vi "FRCts20_Backend_Test_ClosedRequests.vi"(8 "error in (no error)":errorcluster, 11 "Event Name":string) -> (0 "error out":errorcluster, 1 "Time (ms)":u32, 2 "Status":string, 5 "Success":bool)   [LabVIEW 2014, in "FRCts20_Backend_TestCode.lvlib"]
uses:
  FRCts20_Backend_TestCode.lvlib
  FRCts20_Backend_API/FRCts20_Backend_API_ClosedRequests.ctl
  FRCts20_Backend_API/FRCts20_Backend_API_Command_ClosedRequests.ctl
  FRCts20_Backend_API/FRCts20_Backend_API_ClosedRequests.vi
  FRCts20_Backend_API/FRCts20_Backend_API.lvlib
panel:
  out "DataOut":T1
  # "368\n381"
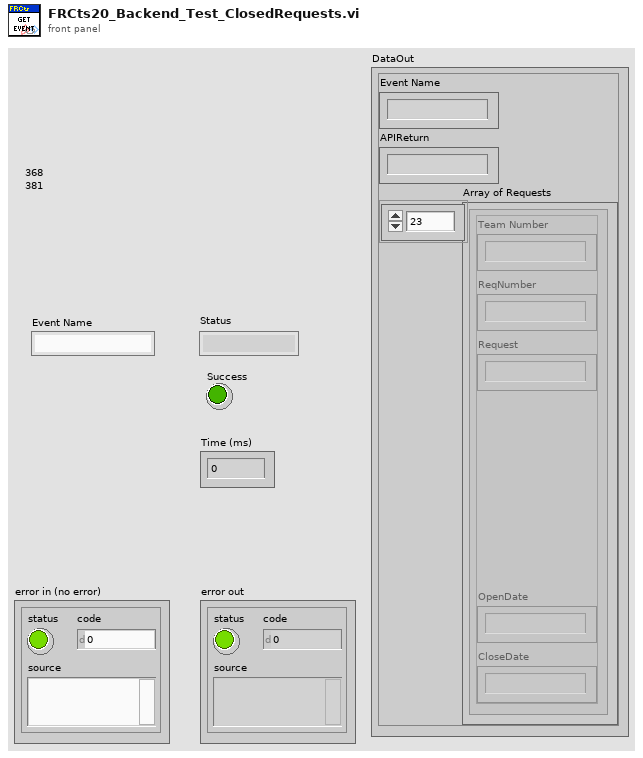
[diagram p1: front panel]
types:
  T1 = typedef "FRCts20_Backend_API.lvlib/FRCts20_Backend_API_ClosedRequests.ctl" = cluster{"Event Name":string, "APIReturn":string, "Array of Requests":cluster{"Team Number":string, "ReqNumber":string, "Request":string, "OpenDate":string, "CloseDate":string}[]}
  T2 = typedef "FRCts20_Backend_API.lvlib/FRCts20_Backend_API_Command_ClosedRequests.ctl" = string
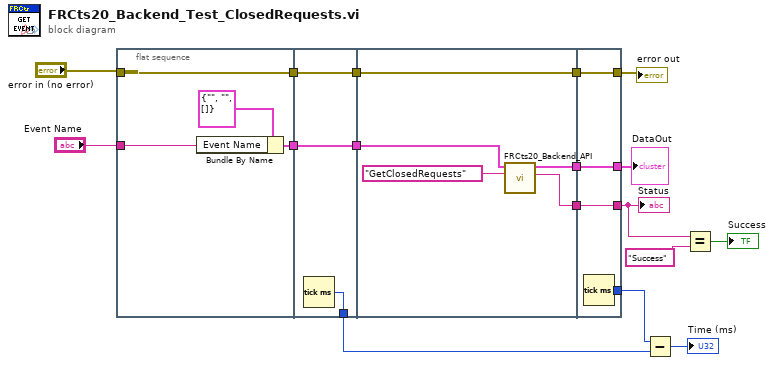
[diagram p0: block diagram]
diagram:
  n1 = flat-sequence {
    tunnel: "error in (no error)" -> [w21]
    tunnel: [w21] -> w15
    tunnel: [w20] -> w3
    tunnel: "Event Name" -> [w19]
    tunnel: [w24] -> w8
    tunnel: [w23] -> w14
    tunnel: w15 -> [w23]
    tunnel: [w22] -> w4
    tunnel: w3 -> [w22]
    tunnel: [w29] -> w13
    tunnel: w14 -> [w29]
    tunnel: [w28] -> w7
    tunnel: [w27] -> w6
    tunnel: w4 -> [w26]
    tunnel: [w33] -> w9
    tunnel: [w32] -> w11
    tunnel: w13 -> [w32]
    tunnel: [w31] -> w1
    tunnel: w7 -> [w31]
    tunnel: [w30] -> w5
    tunnel: w6 -> [w30]
    frame #0 {
      n2 = Bundle By Name(cluster=T1 {"Event Name"="", "APIReturn"="", "Array of Requests"=[]} ("ClosedRequests"), "Event Name"=w19) -> (w20:T1)
    }
    frame #1 {
      n3 = Tick Count (ms)() -> (millisecond timer value=w24:u32)
    }
    frame #2 {
      n4 = call-poly "FRCts20_Backend_API.vi"("Command"=T2 "GetClosedRequests", "DataIn"=w26) -> ("Status"=w27:string, "DataOut"=w28:T1)  [unwired: 7 in, 1 out]
    }
    frame #3 {
      n5 = Tick Count (ms)() -> (millisecond timer value=w33:u32)
    }
  }
  n6 = Subtract(x=w9, y=w8) -> (x-y=→"Time (ms)":u32)
  n7 = Equal?(x=w5, y="Success") -> (x = y?=→"Success":bool)
  "Status" <- w5
  "error out" <- w11
  "DataOut" <- w1
